vi "CRYSequence Generator.vi"() -> ()   [LabVIEW 2013]
uses:
  CRYSystem/Typedef Control/CRYStimulus Type.ctl
  CRYMainGlobal.vi
  CRYSystem/Program/CRYRef nums global.vi
  CRYStepSetup/CRYStepSetup Global.vi
  CRYWindow/SubVI/CRYMain Sub Window Global.vi
  CRYProject/CRYProject Editor Global.vi
  <vilib>/Platform/browser.llb/Open URL in Default Browser (string).vi
panel:
  in  "Save":bool caption="OK"
  in  "Calibrate Microphone":bool caption="OK"
  in  "Save Path":path caption="自动保存文件夹路径"
  out "Autosave":bool
  in  "Save Results":bool
  in  "Save Data":bool
  in  "stop":bool
  out "Polarity_Sign":string="+/-"
  in  "Polarity":bool
  in  "Polarity_Limit":dbl=1.0 caption="Std Err" min=1.0 max=6.0 format="%#_6p"
  in  "MoreInfo":bool
  out "Loose Particle_Sign":string="+/-"
  in  "Loose Particle":bool
  in  "Loose Particle_Limit":dbl=1.0 caption="Std Err" min=1.0 max=6.0 format="%#_6p"
  out "Impedance_Sign":string="+/-"
  out "Rub & Buzz_Sign":string="+"
  out "THD_Sign":string="+"
  out "Sensitivity_Sign":string="+/-"
  out "Fundamental_Sign":string="+/-"
  out "MarkImage":bool
  out "Test Setup":bool
  in  "Rub & Buzz":bool
  in  "Impedance":bool
  out "Reminder":bool
  in  "Impedance_Limit":dbl=1.0 caption="Std Err" min=1.0 max=6.0 format="%#_6p"
  in  "Rub & Buzz_Limit":dbl=1.0 caption="Std Err" min=1.0 max=6.0 format="%#_6p"
  in  "THD_Limit":dbl=1.0 caption="Std Err" min=1.0 max=6.0 format="%#_6p"
  in  "Sensitivity_Limit":dbl=1.0 caption="Std Err" min=1.0 max=6.0 format="%#_6p"
  in  "Fundamental_Limit":dbl=1.0 caption="Std Err" min=1.0 max=6.0 format="%#_6p"
  out "Results":bool
  in  "Test Level(V)":dbl=1.0 min=3.355e-21 max=1.84838 format="%-#1.3p"
  in  "Sweep Time(s)":dbl=1.0 format="%#.3p"
  in  "Start Freq.(Hz)":dbl=1.0 format="%#.3p"
  in  "StopFreq.(Hz)":dbl=1.0 format="%#.3p"
  in  "Sensitivity":bool
  in  "Fundamental":bool
  in  "THD":bool
  in  "OK":bool
  in  "Cancel":bool
  in  "Load Test":bool
  in  "Measure Ref":bool caption="OK"
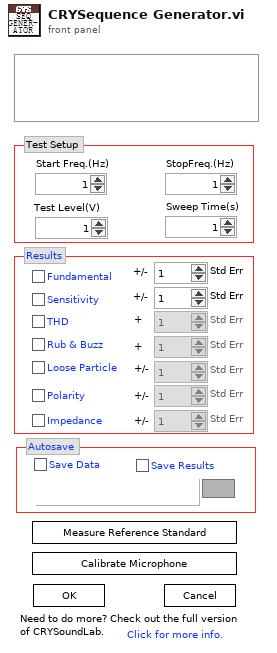
[diagram p1: front panel]
types:
  T1 = enum8{"Enabled", "Disabled", "Disabled and Grayed Out"}
  T2 = enum32{"existing file", "new file", "new or existing file", "existing dir", "new dir", "new or existing dir", "existing file (use LLBs)", "new file (use LLBs)", "new or existing file (use LLBs)", "new or existing file or directory (use LLBs)", "existing dir (use LLBs)", "new dir (use LLBs)", "new or existing dir (use LLBs)", "existing file or dir", "new file or dir", "new or existing file or dir", "existing file or dir (use LLBs)", "new file or dir (use LLBs)"}
  T3 = typedef "CRYStimulus Type.ctl" = u16
  T4 = typedef "CRYTS.ctl" = cluster{"No.TS":u16, "TS File Path":path, "TS Name":string, "EditStepName":string, "Steps":T5[], "New State":bool, "Change State":bool, "Flattened CurveLib Data":string, "Document Data":string, "EditStepNo":u16, "Operator Start File":string, "Sequence Type":string, "Sequence Language":string}
  T5 = typedef "CRYStep.ctl" = cluster{"No.VI":i32, "Category":string, "StepName":string, "Seq setup flattened":string, "Comment":string, "Steps config.":bool[], "Jump config":i32[], "Start":dbl, "Increment":dbl, "Name":string, "Unit":string, "Y data":u16, "Y prefix":string, "Y dB ref":dbl, "Y unit":string, "Repeat State Array":cluster{"Start":dbl, "Increment":dbl, "Count":i32, "Num":i32}[]}
  T6 = typedef "CRYStimulus Cluster.ctl" = cluster{"StimulusType":string, "UseMLValArray":u16[], "ML_axisArray":u16[], "MLValLevelNameArray":string[], "Level(U)Array":dbl[], "Start(Stop)FreqArray":dbl[], "Start(Stop)AmpArray":dbl[], "StepResolutionArray":u16[], "Unit_Array":u16[], "DegValArray":dbl[], "DegUnitArray":string[], "Steps1":i32, "Cycle/step1(#)":u32, "Time/step1(s)":dbl, "Transition1":dbl, "SweepRate2":dbl, "Freq3(Hz)":dbl, "Steps3(#)":dbl, "Cycles3(#)":u32, "StepSize3":dbl, "wave time":string, "RMS_Value4":dbl, "Peak_Value4":dbl, "WavePath4":string, "RMS_unit4":string, "Peak_unit4":string, "wave Info":string, "dc_ctrl5_1":u16, "dc_ctrl5_2":u16, "dc_polar5":u16, "Max.Current":u16, "Steps5(#)":u32, "Time/Step5":dbl, "Level5":dbl, "StepsSize5Val":dbl, "StepSize5Unit":string, "SweepType":u16, "Fixed/Ratio6":u16, "Transition6":dbl, "Steps6(#)":dbl, "Cycle/Steps6(#)":u32, "Time/Steps6(s)":dbl, "Freq6(Hz)":dbl, "Difference6(Hz)":dbl, "Ratio6":string, "NoiseType7":u16, "Duration7(s)":dbl, "MinFreq7(Hz)":dbl, "MaxFreq7(Hz)":dbl, "MinFreq8(Hz)":dbl, "MaxFreq8(Hz)":dbl, "FreqRounding8":bool, "Duration8(s)":dbl, "Tones8":dbl, "RoundingVal8":dbl, "ApplyEQ":bool, "Duration(s)":dbl, "CustomStimulusName ":string, "Flatten Element Array":string[], "sine waves":cluster{"freq":dbl, "ampl":dbl, "cycles":dbl}[], "Channel Out":i32, "RatioVal6":dbl, "TabCtrl6":enum32{"Master Tone", "Slave Tone"}, "Signal Type Name":string, "Help":string, "Channel Sel":u16}
  T7 = typedef "CRYfstepsw.ctl" = cluster{"Level(U)":dbl, "Start Freq(Hz)":dbl, "Stop Freq(Hz)":dbl, "ML val level name":string, "Use ML Val level?":bool, "ML axis":u8, "Steps (#)":i32, "Cycles/step(#)":u32, "Time/step (s)":dbl, "Step Resolution":u16, "unit":u16, "Start Freq Name":string, "Stop Freq Name":string, "Start Freq Axis":u8, "Stop Freq Axis":u8, "Start Freq Flag":string, "Stop Freq Flag":string}
  T8 = typedef "CRYflogsw.ctl" = cluster{"Level(U)":dbl, "Start Freq(Hz)":dbl, "Stop Freq(Hz)":dbl, "Sweep Rate(s/dec)":dbl, "Use ML Val level?":bool, "ML val level name":string, "ML axis":u8, "TSR params":cluster{"FSamp":dbl, "FStart":dbl, "FStop":dbl, "NOffset":dbl, "MStop":dbl, "MStart":dbl, "NHarm":dbl, "Tsamp":dbl, "Amplit":dbl}, "unit":u16, "Start Freq Name":string, "Stop Freq Name":string, "Start Freq Axis":u8, "Stop Freq Axis":u8, "Start Freq Flag":string, "Stop Freq Flag":string}
  T9 = typedef "CRYampsw.ctl" = cluster{"Freq(Hz)":dbl, "Steps (#)":i32, "Cycles(#)":u32, "Use ML Val freq?":bool, "ML val freq name":string, "ML axis":u8, "Start Ampl(U)":dbl, "Stop Ampl(U)":dbl, "unit":u16}
  T10 = typedef "CRYwavefile.ctl" = cluster{"Level(U)":dbl, "Wave Path":string, "ML axis":u8, "ML val level name":string, "Use ML Val level?":bool, "wave info":string, "wave time":string, "Peak value4":dbl, "RMS value4":dbl, "wave channel":u16, "unit":u16}
  T11 = typedef "CRYdcconn.ctl" = cluster{"dc ctrl":u16, "dcmax I":u16, "dc polar":u16, "dc ctrl":u16, "Steps (#)":i32, "Time/step (s)":dbl, "Start Ampl(U)":dbl, "Stop Ampl(U)":dbl, "Level(U)":dbl, "Step Size":dbl}
  T12 = typedef "CRYtwotone.ctl" = cluster{"Steps (#)":i32, "Tone Type":u8, "Freq2(Hz)":dbl, "Time/step (s)":dbl, "Cycles/step (#)":u32, "ML val level name":string, "Use ML Val level?":bool, "Level(U) 2":dbl, "Diff Freq(Hz)":dbl, "ML axis 2":u8, "Diff/Ratio":u8, "Level(U)":dbl, "Stop Freq(Hz)":dbl, "Ratio Val":dbl, "ML val level name 2":string, "Use ML Val level? 2":bool, "ML axis":u8, "Start Freq(Hz)":dbl, "Step Resolution":u16, "Ratio":u16, "TabCtrl6":enum32{"Master Tone", "Slave Tone"}, "unit 1":u16, "unit 2":u16, "Start Freq Name":string, "Stop Freq Name":string, "Start Freq Axis":u8, "Stop Freq Axis":u8, "Start Freq Flag":string, "Stop Freq Flag":string}
  T13 = typedef "CRYmltitone.ctl" = cluster{"Level(U)":dbl, "Min Freq(Hz)":dbl, "Max Freq(Hz)":dbl, "Duration(s)":dbl, "Freq Rounding":bool, "Rounding Val":dbl, "Profile":i32, "ML axis 2":u8, "ML val level name":string, "Use ML Val level?":bool, "ML axis":u8, "Step Resolution":u16, "unit":u16, "Start Freq Name":string, "Stop Freq Name":string, "Start Freq Axis":u8, "Stop Freq Axis":u8, "Start Freq Flag":string, "Stop Freq Flag":string}
  T14 = typedef "CRYnoise.ctl" = cluster{"Noise Type":u8, "Min Freq(Hz)":dbl, "Max Freq(Hz)":dbl, "Level(U)":dbl, "Duration(s)":dbl, "ML val level name":string, "Use ML Val level?":bool, "ML axis":u8, "unit":u16, "Start Freq Name":string, "Stop Freq Name":string, "Start Freq Axis":u8, "Stop Freq Axis":u8, "Start Freq Flag":string, "Stop Freq Flag":string}
  T15 = cluster{"fstepsw":T7, "flogsw":T8, "ampsw":T9, "wavefile":T10, "dcconn":T11, "twotone":T12, "mltitone":T13, "noise":T14, "sqwvsw":cluster{"Level(U)":dbl, "Duty Cycle":dbl, "ML val level name":string, "ML axis":u8, "Start Freq(Hz)":u32, "Stop Freq(Hz)":u32, "Use ML Val level?":bool, "Steps (#)":u32, "Cycles/step (#)":u32, "Time/step (s)":dbl, "Step Resolution":u16}, "tnbrst":cluster{"Level(U)":dbl, "ML val level name":string, "ML axis":u8, "Start Freq(Hz)":u32, "Use ML Val level?":bool, "Cycles/step (#)":u32, "Duration(s)":dbl}}
  T16 = typedef "CRYLimits.ctl" = cluster{"Name":string, "Tolerance":u16, "X Axis":u16, "Limits":u16, "Upper Limit":cluster{dbl, dbl}[], "Align Ref":cluster{dbl, dbl}, "Lower Limit":cluster{dbl, dbl}[], "Y data":u16, "Y unit":string, "Y dB ref":dbl, "Curve Names":string[], "Y-Resolution":u8, "Type":u16, "x float":bool, "X min-max-step":cluster{"Limit X Offset Min":dbl, "Limit X Offset Max":dbl, "Limit X Offset Step Size":dbl}, "magn/phase":u16, "Upper Limit Type":u16, "Lower Limit Type":u16, "Lim Curve axis up":u16, "Lim Curve axis lo":u16, "Data Selection Upper":u16, "Data Selection Lower":u16, "X-Resolution":u8, "Output failed point curves?":bool, "X data":u16, "X unit":string, "X dB ref":dbl, "X-Y Graph Set-up":string, "Tab Value":enum32{"Data", "Parameters"}, "Help":string, "X Up Val":dbl, "Y Up Val":dbl, "X Low Val":dbl, "Y Low Val":dbl, "Up Limit Val":dbl, "Low Limit Val":dbl}
  T17 = enum32{"Invalid", "Standard", "Closed", "Hidden", "Minimized", "Maximized"}
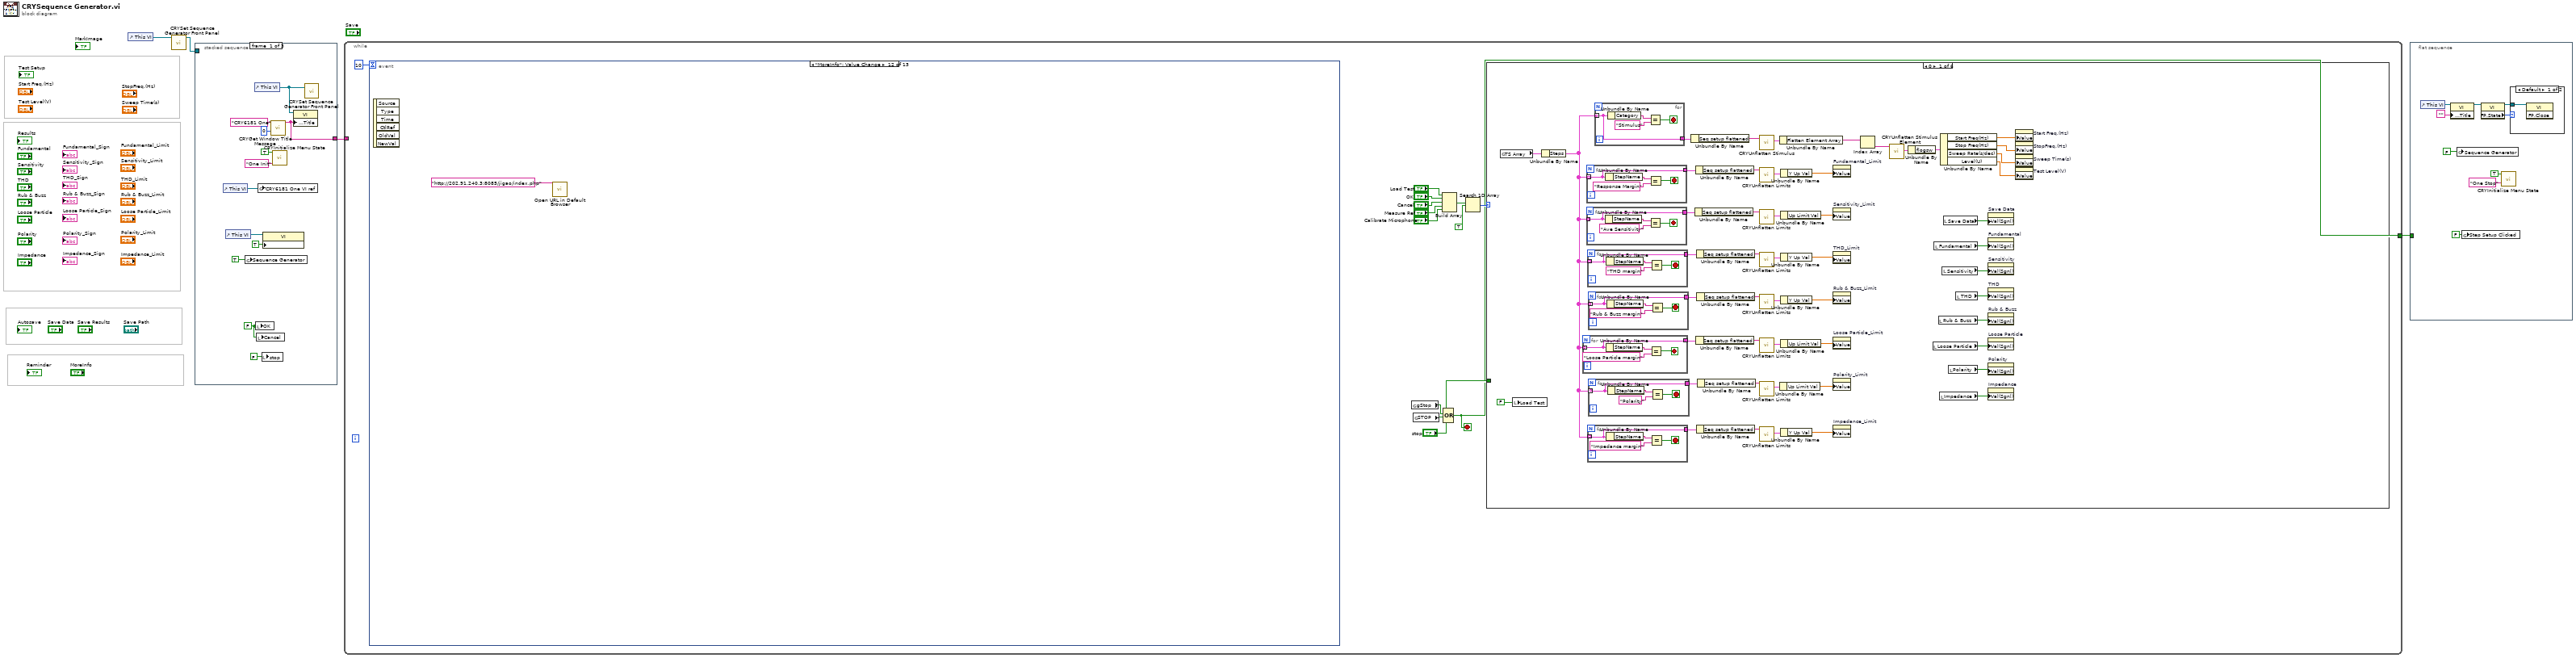
[diagram p0: block diagram]
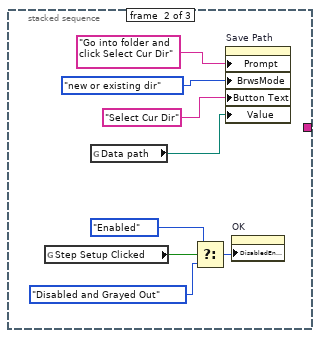
[diagram p3: hidden frame]
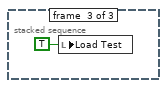
[diagram p4: hidden frame]
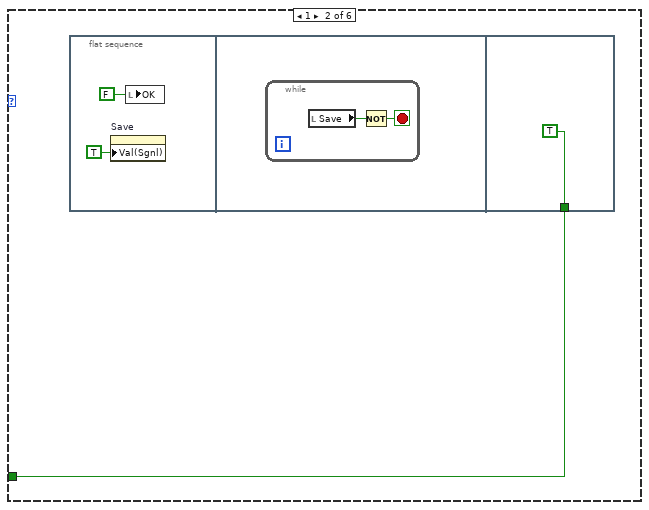
[diagram p5: hidden frame]
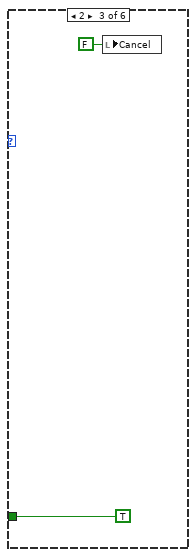
[diagram p6: hidden frame]
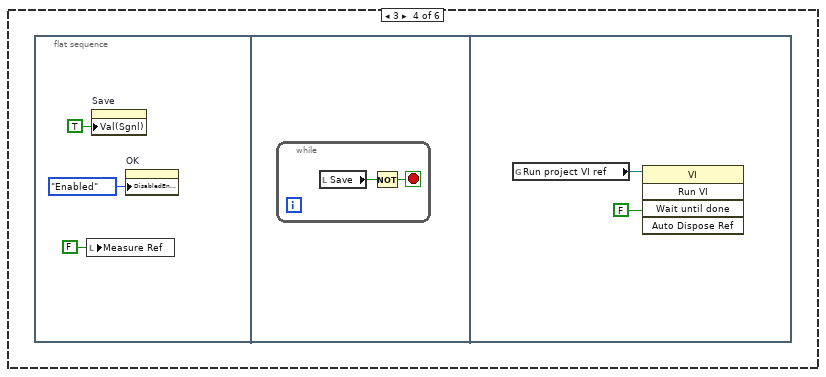
[diagram p7: hidden frame]
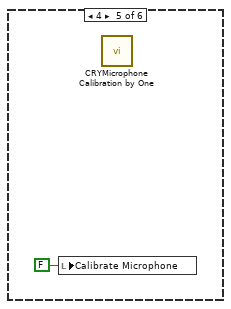
[diagram p8: hidden frame]
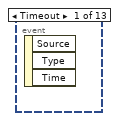
[diagram p10: hidden frame]
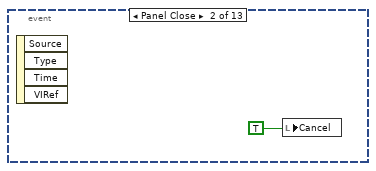
[diagram p11: hidden frame]
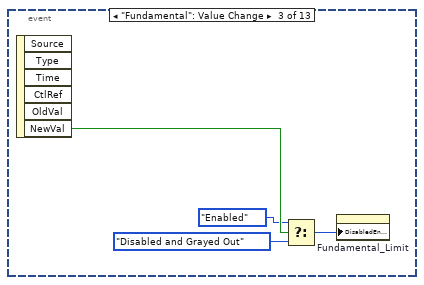
[diagram p12: hidden frame]
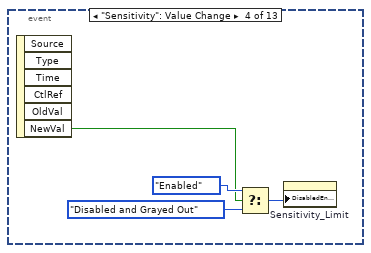
[diagram p13: hidden frame]
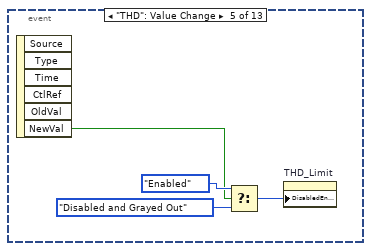
[diagram p14: hidden frame]
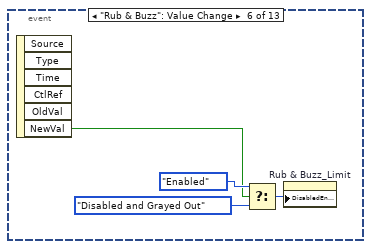
[diagram p15: hidden frame]
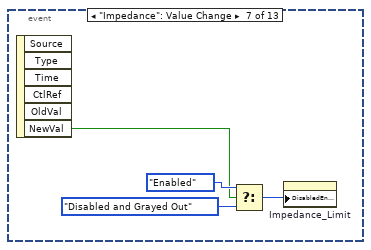
[diagram p16: hidden frame]
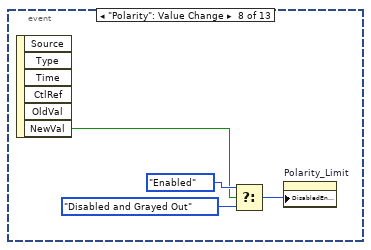
[diagram p17: hidden frame]
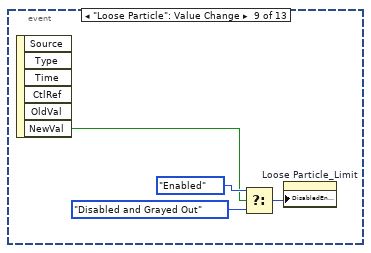
[diagram p18: hidden frame]
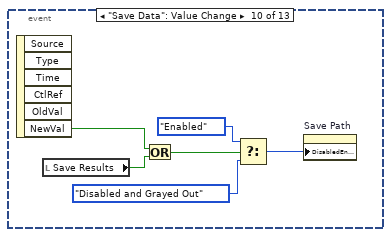
[diagram p19: hidden frame]
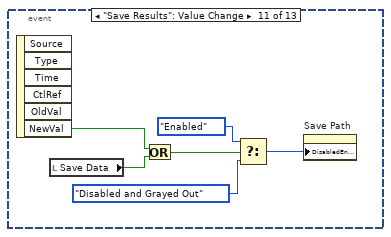
[diagram p20: hidden frame]
diagram:
  n1 = control-ref of="This VI"() -> (w2:refnum<vi>)
  n2 = call "CRYSet Sequence Generator Front Panel.vi"("Vi Ref In"=w2) -> ("Vi Ref Out"=w1:refnum<vi>)  [unwired: 10 in]
  n3 = stacked-sequence {
    tunnel: [w13 _ _] -> w4
    tunnel: w1 -> [_ _ _]
    frame #0 {
      w12 = FALSE ("OK")
      n4 = control-ref of="This VI"() -> (w11:refnum<vi>)
      n5 = control-ref of="This VI"() -> (w9:refnum<vi>)
      n6 = global write "CRYMainGlobal.vi" "Sequence Generator"(TRUE ("Quick Lunch")) -> ()
      n7 = control-ref of="This VI"() -> (w16:refnum<vi>)
      n8 = local write "OK"(w12) -> ()
      n9 = local write "Cancel"(w12) -> ()
      n10 = global write "CRYRef nums global.vi" "CRY6181 One VI ref"(w11) -> ()
      n11 = local write "stop"(FALSE ("stop")) -> ()
      n12 = property class="VI"(reference=w9, "Front Panel.IsFrontmost"=TRUE ("Front Panel Window:Is Frontmost")) -> ()  [unwired: 1 in, 2 out]
      n13 = call "CRYGet Window Title Message.vi"("No"=0 ("Error No"), "Kind"="CRY6181 One") -> ("Multibyte String"=w13:string)  [unwired: 4 in, 5 out]
      n14 = call "CRYInitialize Menu State.vi"("sAction"="One Init", "Is Disable?"=TRUE) -> ()  [unwired: 10 out]
      n15 = property class="VI"(reference=w16, "Front Panel.Title"=w13) -> ()  [unwired: 1 in, 2 out]
      n16 = call "CRYSet Sequence Generator Front Panel.vi"("Vi Ref In"=w16) -> ()  [unwired: 10 in, 1 out]
    }
    frame #1 {
      n17 = global read "CRYStepSetup Global.vi" "Step Setup Clicked"() -> (w20:bool)
      n18 = global read "CRYMainGlobal.vi" "Data path"() -> (w21:path)
      n19 = Select(t=T1."Enabled", s=w20, f=T1."Disabled and Grayed Out" ("Disabled")) -> (s? t:f=w19:T1)
      n20 = property on="Save Path" class="Path"("Prompt"="Go into folder and click Select Cur Dir" ("prompt"), "BrwsMode"=T2."new or existing dir" ("Browse Options:Selection Mode"), "Button Text"="Select Cur Dir" ("Browse Options:Button Text"), "Value"=w21) -> ()  [unwired: 2 in, 2 out]
      n21 = property on="OK" class="Bool (strict)"("DisabledEnum"=w19) -> ()  [unwired: 2 in, 2 out]
    }
    frame #2 {
      n22 = local write "Load Test"(TRUE ("Load Test")) -> ()
    }
  }
  n23 = while {
    tunnel: w4 -> [_]
    tunnel: [w28] -> w3
    stop <- w28 stop-if-true
    n24 = event shown="[11] \"MoreInfo\": Value Change" {
      selector: _ -> [_ _ _ _ _ _ _ _ _ _ _ _ _]
      dyn-events: _ -> [_ _ _ _ _ _ _ _ _ _ _ _ _]
      timeout: 10 -> [_ _ _ _ _ _ _ _ _ _ _ _ _]
      event Timeout {
        n25 = event-data() -> ()  [unwired: 1 in, 3 out]
      }
      event Panel Close {
        n26 = event-data() -> ()  [unwired: 1 in, 4 out]
        n27 = local write "Cancel"(TRUE) -> ()
      }
      event "Fundamental": Value Change {
        n28 = event-data() -> ("NewVal"=w142:bool)  [unwired: 1 in, 5 out]
        n29 = Select(t=T1."Enabled" ("Disabled"), s=w142, f=T1."Disabled and Grayed Out") -> (s? t:f=w139:T1)
        n30 = property on="Fundamental_Limit" class="DigNum (strict)"("DisabledEnum"=w139) -> ()  [unwired: 2 in, 2 out]
      }
      event "Sensitivity": Value Change {
        n31 = event-data() -> ("NewVal"=w144:bool)  [unwired: 1 in, 5 out]
        n32 = Select(t=T1."Enabled" ("Disabled"), s=w144, f=T1."Disabled and Grayed Out") -> (s? t:f=w143:T1)
        n33 = property on="Sensitivity_Limit" class="DigNum (strict)"("DisabledEnum"=w143) -> ()  [unwired: 2 in, 2 out]
      }
      event "THD": Value Change {
        n34 = event-data() -> ("NewVal"=w148:bool)  [unwired: 1 in, 5 out]
        n35 = Select(t=T1."Enabled" ("Disabled"), s=w148, f=T1."Disabled and Grayed Out") -> (s? t:f=w147:T1)
        n36 = property on="THD_Limit" class="DigNum (strict)"("DisabledEnum"=w147) -> ()  [unwired: 2 in, 2 out]
      }
      event "Rub & Buzz": Value Change {
        n37 = event-data() -> ("NewVal"=w152:bool)  [unwired: 1 in, 5 out]
        n38 = Select(t=T1."Enabled" ("Disabled"), s=w152, f=T1."Disabled and Grayed Out") -> (s? t:f=w151:T1)
        n39 = property on="Rub & Buzz_Limit" class="DigNum (strict)"("DisabledEnum"=w151) -> ()  [unwired: 2 in, 2 out]
      }
      event "Impedance": Value Change {
        n40 = event-data() -> ("NewVal"=w156:bool)  [unwired: 1 in, 5 out]
        n41 = Select(t=T1."Enabled" ("Disabled"), s=w156, f=T1."Disabled and Grayed Out") -> (s? t:f=w155:T1)
        n42 = property on="Impedance_Limit" class="DigNum (strict)"("DisabledEnum"=w155) -> ()  [unwired: 2 in, 2 out]
      }
      event "Polarity": Value Change {
        n43 = event-data() -> ("NewVal"=w160:bool)  [unwired: 1 in, 5 out]
        n44 = Select(t=T1."Enabled" ("Disabled"), s=w160, f=T1."Disabled and Grayed Out") -> (s? t:f=w159:T1)
        n45 = property on="Polarity_Limit" class="DigNum (strict)"("DisabledEnum"=w159) -> ()  [unwired: 2 in, 2 out]
      }
      event "Loose Particle": Value Change {
        n46 = event-data() -> ("NewVal"=w164:bool)  [unwired: 1 in, 5 out]
        n47 = Select(t=T1."Enabled" ("Disabled"), s=w164, f=T1."Disabled and Grayed Out") -> (s? t:f=w163:T1)
        n48 = property on="Loose Particle_Limit" class="DigNum (strict)"("DisabledEnum"=w163) -> ()  [unwired: 2 in, 2 out]
      }
      event "Save Data": Value Change {
        n49 = event-data() -> ("NewVal"=w171:bool)  [unwired: 1 in, 5 out]
        n50 = local read "Save Results"() -> (w172:bool)
        n51 = Or(x=w171, y=w172) -> (x .or. y?=w170:bool)
        n52 = Select(t=T1."Enabled" ("Disabled"), s=w170, f=T1."Disabled and Grayed Out") -> (s? t:f=w168:T1)
        n53 = property on="Save Path" class="Path"("DisabledEnum"=w168) -> ()  [unwired: 2 in, 2 out]
      }
      event "Save Results": Value Change {
        n54 = event-data() -> ("NewVal"=w177:bool)  [unwired: 1 in, 5 out]
        n55 = local read "Save Data"() -> (w178:bool)
        n56 = Or(x=w177, y=w178) -> (x .or. y?=w176:bool)
        n57 = Select(t=T1."Enabled" ("Disabled"), s=w176, f=T1."Disabled and Grayed Out") -> (s? t:f=w174:T1)
        n58 = property on="Save Path" class="Path"("DisabledEnum"=w174) -> ()  [unwired: 2 in, 2 out]
      }
      event "MoreInfo": Value Change {
        n59 = event-data() -> ()  [unwired: 1 in, 6 out]
        n60 = call-poly <vilib>:"Open URL in Default Browser.vi"("URL"="http://202.91.240.3:8085/jigao/index.php") -> ()  [unwired: 1 in, 6 out]
      }
      event "Save": Value Change {
        n61 = event-data() -> ()  [unwired: 1 in, 6 out]
        n62 = flat-sequence {
          frame #0 {
            w230 = T3 1 items=["Frequency Stepped Sweep", "Frequency Log Sweep", "Log Amplitude Sweep", "WAV", "DC Connect", "Two Tone", "Noise", "Multitone"] ("Stimulus Type")
            n63 = global read "CRYProject Editor Global.vi" "TS Array"() -> (w243:T4)
            n64 = Unbundle By Name(w243) -> ("Steps"=w196:T5[])
            n65 = for {
              tunnel: w196 -> [w318] mode=indexing
              tunnel: [w318] -> w221
              tunnel: [w317] -> w214
              i -> [w317]
              stop <- w315 stop-if-true
              n66 = Unbundle By Name(w318) -> ("StepName"=w316:string)
              n67 = Equal?(x=w316, y="Loose Particle margin") -> (x = y?=w315:bool)
            }
            n68 = for {
              tunnel: w196 -> [w254] mode=indexing
              tunnel: [w254] -> w198
              tunnel: [w253] -> w195
              i -> [w253]
              stop <- w251 stop-if-true
              n69 = Unbundle By Name(w254) -> ("StepName"=w252:string)
              n70 = Equal?(x=w252, y="Save to Data") -> (x = y?=w251:bool)
            }
            n71 = for {
              tunnel: w196 -> [w328] mode=indexing
              tunnel: [w328] -> w223
              tunnel: [w327] -> w218
              i -> [w327]
              stop <- w325 stop-if-true
              n72 = Unbundle By Name(w328) -> ("StepName"=w326:string)
              n73 = Equal?(x=w326, y="THD margin") -> (x = y?=w325:bool)
            }
            n74 = for {
              tunnel: w196 -> [w323] mode=indexing
              tunnel: [w323] -> w222
              tunnel: [w322] -> w216
              i -> [w322]
              stop <- w320 stop-if-true
              n75 = Unbundle By Name(w323) -> ("StepName"=w321:string)
              n76 = Equal?(x=w321, y="Rub & Buzz margin") -> (x = y?=w320:bool)
            }
            n77 = for {
              tunnel: w196 -> [w348] mode=indexing
              tunnel: [w348] -> w197
              tunnel: [w347] -> w194
              i -> [w347]
              stop <- w345 stop-if-true
              n78 = Unbundle By Name(w348) -> ("StepName"=w346:string)
              n79 = Equal?(x=w346, y="Save to Results") -> (x = y?=w345:bool)
            }
            n80 = for {
              tunnel: w196 -> [w308] mode=indexing
              tunnel: [w308] -> w219
              tunnel: [w307] -> w210
              i -> [w307]
              stop <- w305 stop-if-true
              n81 = Unbundle By Name(w308) -> ("StepName"=w306:string)
              n82 = Equal?(x=w306, y="Impedance margin") -> (x = y?=w305:bool)
            }
            n83 = for {
              tunnel: w196 -> [w338] mode=indexing
              tunnel: [w338] -> w227
              tunnel: [w337] -> w229
              i -> [w337]
              stop <- w335 stop-if-true
              n84 = Unbundle By Name(w338) -> ("StepName"=w336:string)
              n85 = Equal?(x=w336, y="Response Margin") -> (x = y?=w335:bool)
            }
            n86 = for {
              tunnel: w196 -> [w333] mode=indexing
              tunnel: [w333] -> w226
              tunnel: [w332] -> w225
              i -> [w332]
              stop <- w330 stop-if-true
              n87 = Unbundle By Name(w333) -> ("StepName"=w331:string)
              n88 = Equal?(x=w331, y="Ave Sensitivity") -> (x = y?=w330:bool)
            }
            n89 = for {
              tunnel: w196 -> [w313] mode=indexing
              tunnel: [w313] -> w220
              tunnel: [w312] -> w212
              i -> [w312]
              stop <- w310 stop-if-true
              n90 = Unbundle By Name(w313) -> ("StepName"=w311:string)
              n91 = Equal?(x=w311, y="Polarity") -> (x = y?=w310:bool)
            }
            n92 = for {
              tunnel: w196 -> [w343] mode=indexing
              tunnel: [w343] -> w245
              tunnel: [w342] -> w208
              i -> [w342]
              stop <- w340 stop-if-true
              n93 = Unbundle By Name(w343) -> ("Category"=w341:string)
              n94 = Equal?(x=w341, y="Stimulus") -> (x = y?=w340:bool)
            }
            n95 = Unbundle By Name(w245) -> ("Seq setup flattened"=w249:string)
            n96 = local read "Loose Particle"() -> (w201:bool)
            n97 = local read "Fundamental"() -> (w205:bool)
            n98 = local read "Sensitivity"() -> (w204:bool)
            n99 = local read "Save Results"() -> (w182:bool)
            n100 = local read "Rub & Buzz"() -> (w202:bool)
            n101 = local read "Impedance"() -> (w199:bool)
            n102 = local read "Save Data"() -> (w191:bool)
            n103 = local read "Polarity"() -> (w200:bool)
            n104 = local read "THD"() -> (w203:bool)
            n105 = call "CRYUnflatten Stimulus.vi"("Flatten Stimulus"=w249) -> ("Stimulus"=w248:T6)  [unwired: 10 out]
            n106 = case shown="True" w205 {
              tunnel: [w297 w302] -> w228
              tunnel: w227 -> [w297 w301]
              frame False {
              }
              frame True {
                n107 = local read "Fundamental_Limit"() -> (w298:dbl)
                n108 = Unbundle By Name(w301) -> ("Seq setup flattened"=w300:string)
                n109 = call "CRYChange Limits Flatten Data by One.vi"("Option"="Response Margin" ("y"), "Value"=w298, "Flatten Limits In"=w300) -> ("Flatten Limits Out"=w303:string)  [unwired: 7 in, 1 out]
                n110 = Bundle By Name(cluster=w301, "Seq setup flattened"=w303) -> (w302:T5)
              }
            }
            n111 = case shown="True" w201 {
              tunnel: w221 -> [w269 w275]
              tunnel: [w269 w272] -> w213
              frame False {
              }
              frame True {
                n112 = Unbundle By Name(w275) -> ("Seq setup flattened"=w274:string)
                n113 = local read "Loose Particle_Limit"() -> (w270:dbl)
                n114 = call "CRYChange Limits Flatten Data by One.vi"("Option"="Loose Particle margin" ("y"), "Value"=w270, "Flatten Limits In"=w274) -> ("Flatten Limits Out"=w273:string)  [unwired: 7 in, 1 out]
                n115 = Bundle By Name(cluster=w275, "Seq setup flattened"=w273) -> (w272:T5)
              }
            }
            n116 = case shown="True" w204 {
              tunnel: w226 -> [w290 w294]
              tunnel: [w290 w293] -> w224
              frame False {
              }
              frame True {
                n117 = Unbundle By Name(w294) -> ("Seq setup flattened"=w295:string)
                n118 = local read "Sensitivity_Limit"() -> (w291:dbl)
                n119 = call "CRYChange Limits Flatten Data by One.vi"("Option"="Ave Sensitivity" ("y"), "Value"=w291, "Flatten Limits In"=w295) -> ("Flatten Limits Out"=w296:string)  [unwired: 7 in, 1 out]
                n120 = Bundle By Name(cluster=w294, "Seq setup flattened"=w296) -> (w293:T5)
              }
            }
            n121 = case shown="True" w200 {
              tunnel: w220 -> [w262 w266]
              tunnel: [w262 w265] -> w211
              frame False {
              }
              frame True {
                n122 = Unbundle By Name(w266) -> ("Seq setup flattened"=w267:string)
                n123 = local read "Polarity_Limit"() -> (w263:dbl)
                n124 = call "CRYChange Limits Flatten Data by One.vi"("Option"="Polarity" ("y"), "Value"=w263, "Flatten Limits In"=w267) -> ("Flatten Limits Out"=w268:string)  [unwired: 7 in, 1 out]
                n125 = Bundle By Name(cluster=w266, "Seq setup flattened"=w268) -> (w265:T5)
              }
            }
            n126 = case shown="True" w199 {
              tunnel: w219 -> [w255 w261]
              tunnel: [w255 w258] -> w209
              frame False {
              }
              frame True {
                n127 = Unbundle By Name(w261) -> ("Seq setup flattened"=w260:string)
                n128 = local read "Impedance_Limit"() -> (w256:dbl)
                n129 = call "CRYChange Limits Flatten Data by One.vi"("Option"="Impedance margin" ("y"), "Value"=w256, "Flatten Limits In"=w260) -> ("Flatten Limits Out"=w259:string)  [unwired: 7 in, 1 out]
                n130 = Bundle By Name(cluster=w261, "Seq setup flattened"=w259) -> (w258:T5)
              }
            }
            n131 = case shown="True" w203 {
              tunnel: w223 -> [w283 w289]
              tunnel: [w283 w286] -> w217
              frame False {
              }
              frame True {
                n132 = Unbundle By Name(w289) -> ("Seq setup flattened"=w288:string)
                n133 = local read "THD_Limit"() -> (w284:dbl)
                n134 = call "CRYChange Limits Flatten Data by One.vi"("Option"="THD margin" ("y"), "Value"=w284, "Flatten Limits In"=w288) -> ("Flatten Limits Out"=w287:string)  [unwired: 7 in, 1 out]
                n135 = Bundle By Name(cluster=w289, "Seq setup flattened"=w287) -> (w286:T5)
              }
            }
            n136 = case shown="True" w202 {
              tunnel: w222 -> [w276 w280]
              tunnel: [w276 w279] -> w215
              frame False {
              }
              frame True {
                n137 = Unbundle By Name(w280) -> ("Seq setup flattened"=w281:string)
                n138 = local read "Rub & Buzz_Limit"() -> (w277:dbl)
                n139 = call "CRYChange Limits Flatten Data by One.vi"("Option"="Rub & Buzz margin" ("y"), "Value"=w277, "Flatten Limits In"=w281) -> ("Flatten Limits Out"=w282:string)  [unwired: 7 in, 1 out]
                n140 = Bundle By Name(cluster=w280, "Seq setup flattened"=w282) -> (w279:T5)
              }
            }
            n141 = Unbundle By Name(w248) -> ("Flatten Element Array"=w233:string[])
            n142 = Select(t="Save to Data" ("y"), s=w191, f="No Save to Data" ("y")) -> (s? t:f=w181:string)
            n143 = Select(t="Save to Results" ("y"), s=w182, f="No Save to Results" ("y")) -> (s? t:f=w180:string)
            n144 = property on="Start Freq.(Hz)" class="DigNum (strict)"() -> ("Value"=w237:dbl)  [unwired: 2 in, 2 out]
            n145 = property on="StopFreq.(Hz)" class="DigNum (strict)"() -> ("Value"=w236:dbl)  [unwired: 2 in, 2 out]
            n146 = property on="Test Level(V)" class="DigNum (strict)"() -> ("Value"=w235:dbl)  [unwired: 2 in, 2 out]
            n147 = property on="Sweep Time(s)" class="DigNum (strict)"() -> ("Value"=w234:dbl)  [unwired: 2 in, 2 out]
            n148 = Index Array(array=w233) -> (element=w242:string)  [unwired: 1 in]
            n149 = call "CRYUnflatten Stimulus Element.vi"("Unflatten Stimulus Element setup"=w242) -> ("Stimulus Default"=w241:T15)  [unwired: 1 in, 9 out]
            n150 = Unbundle By Name(w198) -> ("Seq setup flattened"=w190:string)
            n151 = Unbundle By Name(w197) -> ("Seq setup flattened"=w188:string)
            n152 = Unbundle By Name(w241) -> ("flogsw"=w240:T8)
            n153 = Bundle By Name(cluster=w240, "Start Freq(Hz)"=w237, "Stop Freq(Hz)"=w236, "Level(U)"=w235, "Sweep Rate(s/dec)"=w234) -> (w239:T8)
            n154 = Variant To Flattened String(Variant=w239) -> (data string=w238:string)  [unwired: 1 out]
            n155 = call "CRYChange Autosave Flatten Data by One.vi"("Option"=w181, "Flatten Autosave In"=w190) -> ("Flatten Autosave Out"=w189:string)  [unwired: 9 in]
            n156 = call "CRYChange Autosave Flatten Data by One.vi"("Option"=w180, "Flatten Autosave In"=w188) -> ("Flatten Autosave Out"=w187:string)  [unwired: 9 in]
            n157 = call "CRYFlatten Stimulus Element.vi"("Stimulus Type"=w230, "Flattened Stimulus Element"=w238) -> ("Flatten Stimulus Setup String"=w232:string)  [unwired: 9 in]
            n158 = Build Array(w232) -> (w231:string[])
            n159 = Bundle By Name(cluster=w248, "Flatten Element Array"=w231) -> (w247:T6)
            n160 = Bundle By Name(cluster=w198, "Seq setup flattened"=w189) -> (w193:T5)
            n161 = Bundle By Name(cluster=w197, "Seq setup flattened"=w187) -> (w192:T5)
            n162 = call "CRYFlatten Stimulus.vi"("Stimulus"=w247) -> ("Flatten Stimulus String"=w246:string)  [unwired: 10 in]
            n163 = Bundle By Name(cluster=w245, "Seq setup flattened"=w246) -> (w207:T5)
            n164 = Replace Array Subset(array=w196, new element #1=w207, index #1=w208, new element #2=w228, index #2=w229, new element #3=w224, index #3=w225, new element #4=w217, index #4=w218, new element #5=w215, index #5=w216, new element #6=w213, index #6=w214, new element #7=w211, index #7=w212, new element #8=w209, index #8=w210, new element #9=w193, index #9=w195, new element #10=w192, index #10=w194) -> (w206:T5[])
            n165 = Bundle By Name(cluster=w243, "Steps"=w206) -> (w244:T4)
            n166 = global write "CRYProject Editor Global.vi" "TS Array"(w244) -> ()
          }
          frame #1 {
            n167 = local write "Save"(FALSE ("Save")) -> ()
          }
        }
      }
    }
    n168 = global read "CRYMain Sub Window Global.vi" "gStop"() -> (w33:bool)
    n169 = global read "CRYMainGlobal.vi" "STOP"() -> (w32:bool)
    n170 = Build Array("Load Test", "OK", "Cancel", "Measure Ref", "Calibrate Microphone") -> (w37:bool[])
    n171 = Search 1D Array(1D array=w37, element=TRUE) -> (index of element=w35:i32)  [unwired: 1 out]
    n172 = case shown="0" w35 {
      tunnel: [_ w122 TRUE ("Cancel") _ _ _] -> w29
      frame 0 {
        n173 = global read "CRYProject Editor Global.vi" "TS Array"() -> (w85:T4)
        n174 = local write "Load Test"(FALSE ("Cancel")) -> ()
        n175 = Unbundle By Name(w85) -> ("Steps"=w54:T5[])
        n176 = for {
          tunnel: w54 -> [w101] mode=indexing
          tunnel: [w101] -> w63
          stop <- w99 stop-if-true
          n177 = Unbundle By Name(w101) -> ("StepName"=w100:string)
          n178 = Equal?(x=w100, y="Loose Particle margin") -> (x = y?=w99:bool)
        }
        n179 = for {
          tunnel: w54 -> [w113] mode=indexing
          tunnel: [w113] -> w70
          stop <- w111 stop-if-true
          n180 = Unbundle By Name(w113) -> ("StepName"=w112:string)
          n181 = Equal?(x=w112, y="Ave Sensitivity") -> (x = y?=w111:bool)
        }
        n182 = for {
          tunnel: w54 -> [w117] mode=indexing
          tunnel: [w117] -> w81
          stop <- w115 stop-if-true
          n183 = Unbundle By Name(w117) -> ("StepName"=w116:string)
          n184 = Equal?(x=w116, y="Response Margin") -> (x = y?=w115:bool)
        }
        n185 = for {
          tunnel: w54 -> [w109] mode=indexing
          tunnel: [w109] -> w69
          stop <- w107 stop-if-true
          n186 = Unbundle By Name(w109) -> ("StepName"=w108:string)
          n187 = Equal?(x=w108, y="THD margin") -> (x = y?=w107:bool)
        }
        n188 = for {
          tunnel: w54 -> [w93] mode=indexing
          tunnel: [w93] -> w57
          stop <- w91 stop-if-true
          n189 = Unbundle By Name(w93) -> ("StepName"=w92:string)
          n190 = Equal?(x=w92, y="Impedance margin") -> (x = y?=w91:bool)
        }
        n191 = for {
          tunnel: w54 -> [w105] mode=indexing
          tunnel: [w105] -> w64
          stop <- w103 stop-if-true
          n192 = Unbundle By Name(w105) -> ("StepName"=w104:string)
          n193 = Equal?(x=w104, y="Rub & Buzz margin") -> (x = y?=w103:bool)
        }
        n194 = for {
          tunnel: w54 -> [w97] mode=indexing
          tunnel: [w97] -> w58
          stop <- w95 stop-if-true
          n195 = Unbundle By Name(w97) -> ("StepName"=w96:string)
          n196 = Equal?(x=w96, y="Polarity") -> (x = y?=w95:bool)
        }
        n197 = for {
          tunnel: w54 -> [w121] mode=indexing
          tunnel: [w121] -> w86
          stop <- w119 stop-if-true
          n198 = Unbundle By Name(w121) -> ("Category"=w120:string)
          n199 = Equal?(x=w120, y="Stimulus") -> (x = y?=w119:bool)
        }
        n200 = Unbundle By Name(w86) -> ("Seq setup flattened"=w88:string)
        n201 = Unbundle By Name(w70) -> ("Seq setup flattened"=w71:string)
        n202 = Unbundle By Name(w81) -> ("Seq setup flattened"=w80:string)
        n203 = Unbundle By Name(w63) -> ("Seq setup flattened"=w62:string)
        n204 = Unbundle By Name(w69) -> ("Seq setup flattened"=w68:string)
        n205 = Unbundle By Name(w57) -> ("Seq setup flattened"=w56:string)
        n206 = Unbundle By Name(w64) -> ("Seq setup flattened"=w65:string)
        n207 = Unbundle By Name(w58) -> ("Seq setup flattened"=w59:string)
        n208 = call "CRYUnflatten Stimulus.vi"("Flatten Stimulus"=w88) -> ("Stimulus"=w87:T6)  [unwired: 10 out]
        n209 = call "CRYUnflatten Limits.vi"("Unflatten Limits"=w80) -> ("Limits"=w74:T16)  [unwired: 8 in, 2 out]
        n210 = call "CRYUnflatten Limits.vi"("Unflatten Limits"=w71) -> ("Limits"=w72:T16)  [unwired: 8 in, 2 out]
        n211 = call "CRYUnflatten Limits.vi"("Unflatten Limits"=w68) -> ("Limits"=w67:T16)  [unwired: 8 in, 2 out]
        n212 = call "CRYUnflatten Limits.vi"("Unflatten Limits"=w65) -> ("Limits"=w66:T16)  [unwired: 8 in, 2 out]
        n213 = call "CRYUnflatten Limits.vi"("Unflatten Limits"=w62) -> ("Limits"=w61:T16)  [unwired: 8 in, 2 out]
        n214 = call "CRYUnflatten Limits.vi"("Unflatten Limits"=w59) -> ("Limits"=w60:T16)  [unwired: 8 in, 2 out]
        n215 = call "CRYUnflatten Limits.vi"("Unflatten Limits"=w56) -> ("Limits"=w55:T16)  [unwired: 8 in, 2 out]
        n216 = Unbundle By Name(w87) -> ("Flatten Element Array"=w82:string[])
        n217 = Unbundle By Name(w60) -> ("Up Limit Val"=w48:dbl)
        n218 = Unbundle By Name(w74) -> ("Y Up Val"=w73:dbl)
        n219 = Unbundle By Name(w72) -> ("Up Limit Val"=w53:dbl)
        n220 = Unbundle By Name(w67) -> ("Y Up Val"=w52:dbl)
        n221 = Unbundle By Name(w66) -> ("Y Up Val"=w51:dbl)
        n222 = Unbundle By Name(w61) -> ("Up Limit Val"=w50:dbl)
        n223 = Unbundle By Name(w55) -> ("Y Up Val"=w49:dbl)
        n224 = property on="Fundamental_Limit" class="DigNum (strict)"("Value"=w73) -> ()  [unwired: 2 in, 2 out]
        n225 = property on="Sensitivity_Limit" class="DigNum (strict)"("Value"=w53) -> ()  [unwired: 2 in, 2 out]
        n226 = property on="THD_Limit" class="DigNum (strict)"("Value"=w52) -> ()  [unwired: 2 in, 2 out]
        n227 = property on="Rub & Buzz_Limit" class="DigNum (strict)"("Value"=w51) -> ()  [unwired: 2 in, 2 out]
        n228 = property on="Loose Particle_Limit" class="DigNum (strict)"("Value"=w50) -> ()  [unwired: 2 in, 2 out]
        n229 = property on="Polarity_Limit" class="DigNum (strict)"("Value"=w48) -> ()  [unwired: 2 in, 2 out]
        n230 = property on="Impedance_Limit" class="DigNum (strict)"("Value"=w49) -> ()  [unwired: 2 in, 2 out]
        n231 = Index Array(array=w82) -> (element=w84:string)  [unwired: 1 in]
        n232 = call "CRYUnflatten Stimulus Element.vi"("Unflatten Stimulus Element setup"=w84) -> ("Stimulus Default"=w83:T15)  [unwired: 1 in, 9 out]
        n233 = Unbundle By Name(w83) -> ("flogsw"=w79:T8)
        n234 = local read "Loose Particle"() -> (w42:bool)
        n235 = local read "Fundamental"() -> (w46:bool)
        n236 = local read "Rub & Buzz"() -> (w43:bool)
        n237 = local read "Impedance"() -> (w40:bool)
        n238 = Unbundle By Name(w79) -> ("Start Freq(Hz)"=w78:dbl, "Stop Freq(Hz)"=w77:dbl, "Sweep Rate(s/dec)"=w76:dbl, "Level(U)"=w75:dbl)
        n239 = local read "Sensitivity"() -> (w45:bool)
        n240 = local read "Save Data"() -> (w47:bool)
        n241 = local read "Polarity"() -> (w41:bool)
        n242 = local read "THD"() -> (w44:bool)
        n243 = property on="Save Data" class="Bool (strict)"("Val(Sgnl)"=w47) -> ()  [unwired: 2 in, 2 out]
        n244 = property on="Fundamental" class="Bool (strict)"("Val(Sgnl)"=w46) -> ()  [unwired: 2 in, 2 out]
        n245 = property on="Sensitivity" class="Bool (strict)"("Val(Sgnl)"=w45) -> ()  [unwired: 2 in, 2 out]
        n246 = property on="THD" class="Bool (strict)"("Val(Sgnl)"=w44) -> ()  [unwired: 2 in, 2 out]
        n247 = property on="Rub & Buzz" class="Bool (strict)"("Val(Sgnl)"=w43) -> ()  [unwired: 2 in, 2 out]
        n248 = property on="Loose Particle" class="Bool (strict)"("Val(Sgnl)"=w42) -> ()  [unwired: 2 in, 2 out]
        n249 = property on="Polarity" class="Bool (strict)"("Val(Sgnl)"=w41) -> ()  [unwired: 2 in, 2 out]
        n250 = property on="Impedance" class="Bool (strict)"("Val(Sgnl)"=w40) -> ()  [unwired: 2 in, 2 out]
        n251 = property on="Start Freq.(Hz)" class="DigNum (strict)"("Value"=w78) -> ()  [unwired: 2 in, 2 out]
        n252 = property on="StopFreq.(Hz)" class="DigNum (strict)"("Value"=w77) -> ()  [unwired: 2 in, 2 out]
        n253 = property on="Sweep Time(s)" class="DigNum (strict)"("Value"=w76) -> ()  [unwired: 2 in, 2 out]
        n254 = property on="Test Level(V)" class="DigNum (strict)"("Value"=w75) -> ()  [unwired: 2 in, 2 out]
      }
      frame 1 {
        n255 = flat-sequence {
          tunnel: [TRUE ("Save")] -> w122
          frame #0 {
            n256 = property on="Save" class="Bool (strict)"("Val(Sgnl)"=TRUE ("Value (Signaling)")) -> ()  [unwired: 2 in, 2 out]
            n257 = local write "OK"(FALSE ("Cancel")) -> ()
          }
          frame #1 {
            n258 = while {
              stop <- w125 stop-if-true
              n259 = local read "Save"() -> (w126:bool)
              n260 = Not(x=w126) -> (.not. x?=w125:bool)
            }
          }
          frame #2 {
          }
        }
      }
      frame 2 {
        n261 = local write "Cancel"(FALSE ("Cancel")) -> ()
      }
      frame 3 {
        n262 = flat-sequence {
          frame #0 {
            n263 = local write "Measure Ref"(FALSE ("Measure Ref")) -> ()
            n264 = property on="Save" class="Bool (strict)"("Val(Sgnl)"=TRUE ("Value (Signaling)")) -> ()  [unwired: 2 in, 2 out]
            n265 = property on="OK" class="Bool (strict)"("DisabledEnum"=T1."Enabled" ("Disabled")) -> ()  [unwired: 2 in, 2 out]
          }
          frame #1 {
            n266 = while {
              stop <- w133 stop-if-true
              n267 = local read "Save"() -> (w134:bool)
              n268 = Not(x=w134) -> (.not. x?=w133:bool)
            }
          }
          frame #2 {
            n269 = global read "CRYRef nums global.vi" "Run project VI ref"() -> (w135:refnum<vi>)
            n270 = invoke class="VI" method="Run VI"(reference=w135, "Wait until done"=FALSE ("Wait Until Done")) -> ()  [unwired: 3 in, 5 out]
          }
        }
      }
      frame 4 {
        n271 = local write "Calibrate Microphone"(FALSE ("Calibrate Microphone")) -> ()
        n272 = call "CRYMicrophone Calibration by One.vi"() -> ()  [unwired: 12 in]
      }
      frame Default {
      }
    }
    n273 = Compound Arithmetic op=OR(w29, w33, w32, "stop") -> (w28:bool)
  }
  n274 = flat-sequence {
    tunnel: w3 -> [_]
    frame #0 {
      n275 = control-ref of="This VI"() -> (w358:refnum<vi>)
      n276 = property class="VI"(reference=w358, "Front Panel.Title"="") -> (reference out=w356:refnum<vi>)  [unwired: 1 in, 1 out]
      n277 = global write "CRYMainGlobal.vi" "Sequence Generator"(FALSE ("Quick Lunch")) -> ()
      n278 = global write "CRYStepSetup Global.vi" "Step Setup Clicked"(FALSE ("Step Step Clicked")) -> ()
      n279 = property class="VI"(reference=w356) -> (reference out=w354:refnum<vi>, "FP.State"=w355:T17)  [unwired: 1 in, 1 out]
      n280 = call "CRYInitialize Menu State.vi"("sAction"="One Stop", "Is Disable?"=TRUE) -> ()  [unwired: 10 in]
      n281 = case shown="Default" w355 {
        tunnel: w354 -> [w359 _]
        frame Default {
          n282 = invoke class="VI" method="FP.Close"(reference=w359) -> ()  [unwired: 2 in, 3 out]
        }
        frame "Closed" {
        }
      }
    }
  }
